vi "난수발생 .vi"() -> ()   [LabVIEW 2014]
panel:
  in  "가운데로":bool
  in  "메뉴바/도구바":bool
  in  "경로":path
  in  "정지":bool
  in  "난수발생":bool
  out "웨이브폼 차트":dbl(graph)
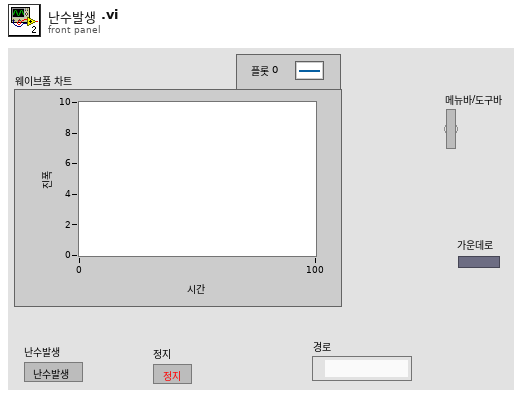
[diagram p1: front panel]
types:
  T1 = enum16{"Always On", "Always Off", "Off While Running"}
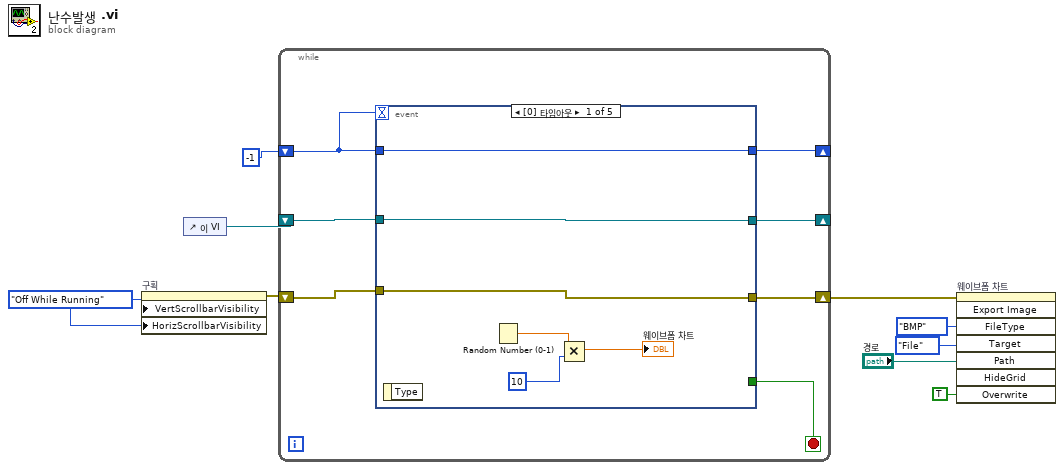
[diagram p0: block diagram]
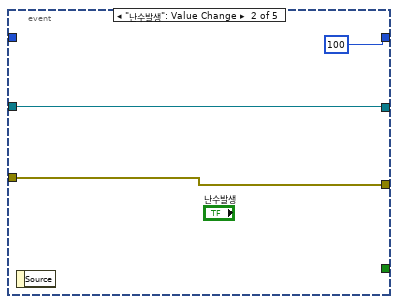
[diagram p2: hidden frame]
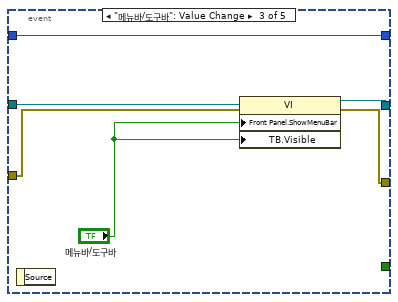
[diagram p3: hidden frame]
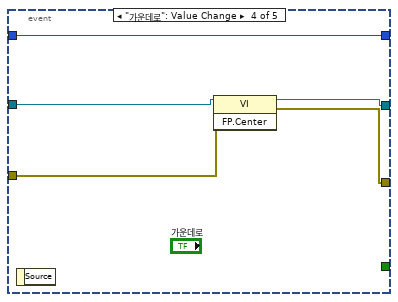
[diagram p4: hidden frame]
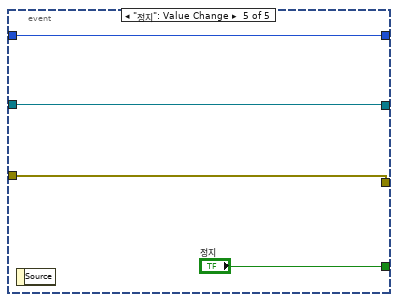
[diagram p5: hidden frame]
diagram:
  w6 = T1."Off While Running" ("수직 스크롤 막대 보이기")
  n1 = property on="구획" class="Pane"("VertScrollbarVisibility"=w6, "HorizScrollbarVisibility"=w6) -> (error out=w7:errorcluster)  [unwired: 2 in, 1 out]
  n2 = control-ref of="이 VI"() -> (w8:refnum<vi>)
  n3 = while {
    shift-right: [w15] -> _
    shift-left: -1 -> [w16]
    shift-right: [w13] -> _
    shift-left: w8 -> [w14]
    shift-right: [w11] -> w5
    shift-left: w7 -> [w12]
    stop <- w10 stop-if-true
    n4 = event shown="[0] 타임아웃" {
      selector: _ -> [_ _ _ _ _]
      dyn-events: _ -> [_ _ _ _ _]
      timeout: w16 -> [_ _ _ _ _]
      tunnel: w16 -> [w19 _ w31 w36 w40]
      tunnel: [w19 100 _ w36 _] -> w15
      tunnel: w14 -> [w18 w24 w30 w35 w39]
      tunnel: [w18 w24 w29 w34 w39] -> w13
      tunnel: w12 -> [w17 w23 w27 w33 w38]
      tunnel: [w17 w23 w28 w32 w38] -> w11
      tunnel: [_ _ w31 _ _] -> _
      tunnel: [_ _ _ _ w40] -> _
      tunnel: [_ _ _ _ "정지"] -> w10
      event Timeout {
        n5 = event-data() -> ()  [unwired: 1 in, 1 out]
        n6 = Random Number (0-1)() -> (number: 0 to 1=w22:dbl)
        n7 = Multiply(x=w22, y=10) -> (x*y=→"웨이브폼 차트":dbl)
      }
      event "난수발생": Value Change {
        n8 = event-data() -> ()  [unwired: 1 in, 1 out]
      }
      event "메뉴바/도구바": Value Change {
        n9 = event-data() -> ()  [unwired: 1 in, 1 out]
        n10 = property class="VI"(reference=w30, error in=w27, "Front Panel.ShowMenuBar"="메뉴바/도구바", "TB.Visible"="메뉴바/도구바") -> (reference out=w29:refnum<vi>, error out=w28:errorcluster)
      }
      event "가운데로": Value Change {
        n11 = event-data() -> ()  [unwired: 1 in, 1 out]
        n12 = invoke class="VI" method="FP.Center"(reference=w35, error in=w33) -> (reference out=w34:refnum<vi>, error out=w32:errorcluster)  [unwired: 1 in, 1 out]
      }
      event "정지": Value Change {
        n13 = event-data() -> ()  [unwired: 1 in, 1 out]
      }
    }
  }
  n14 = invoke on="웨이브폼 차트" class="WFChart (엄격한)" method="Export Image"(error in=w5, "FileType"=enum32{"BMP", "EPS", "EMF", "PICT"}."BMP" ("파일 타입"), "Target"=enum32{"File", "Clipboard"}."File" ("타겟"), "Path"="경로", "Overwrite"=TRUE ("항상 덮어쓰기")) -> ()  [unwired: 3 in, 8 out]
